vi "example_02_convert.vi"() -> ()   [LabVIEW 2015, in "lv-unit-conversion.lvlib"] (continued)
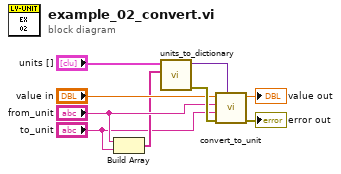
[diagram p0: block diagram]
diagram:
  n1 = Build Array("from_unit", "to_unit") -> (w5:string[])
  n2 = call "units_to_dictionary.vi"("symbols []"=w5, "units []"="units []") -> ("error out"=w9:errorcluster, "unit_set out"=w3:variant)  [unwired: 8 in]
  n3 = call "convert_to_unit.vi"("unit_set"=w3, "error in (no error)"=w9, "unit_to"="to_unit", "unit_from"="from_unit", "value in"="value in") -> ("error out"=→"error out":errorcluster, "value out"=→"value out":dbl)  [unwired: 5 in]
